vi "camera shutter.vi"() -> ()   [LabVIEW 2015]
doc: "Manually blink and LED attached to a digital output channel of a LINX device by clicking and LED control in LabVIEW."
uses:
  <vilib>/MakerHub/LINX/Public/Peripherals/Analog/Analog Read 1 Chan.vi
  <vilib>/MakerHub/LINX/Public/Peripherals/Digital/Digital Write N Chans.vi
  <vilib>/MakerHub/LINX/LMH-LINX.lvlib
panel:
  in  "Analog Channel":u8
  in  "OK Button":bool
  out "Loop Rate (Hz)":u32
  in  "Serial Port":refnum<visa-resource-name>
  in  "Stop Button":bool
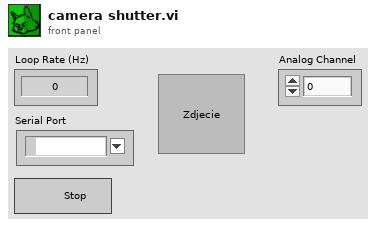
[diagram p1: front panel]
types:
  T1 = typedef "LMH-LINX.lvlib/LINX Ref.ctl" = cluster{"Platform":T2, "Interface":T3, "LINX Device Config":T4}
  T2 = typedef "LMH-LINX.lvlib/Platform.ctl" = enum16{"LINX", "myRIO"}
  T3 = typedef "LMH-LINX.lvlib/Interface.ctl" = enum16{"Serial", "TCP"}
  T4 = typedef "LMH-LINX.lvlib/Device.lvlib/LINX Device Config.ctl" = cluster{"Interface":T3, "COM Port":refnum<visa-resource-name>, "TCP Configuration":T5, "Device Family":u8, "Device ID":u8, "Device Name":string, "TCP Ref":refnum<k5>, "Channels":T6}
  T5 = typedef "LMH-LINX.lvlib/Device.lvlib/TCP Config.ctl" = cluster{"IP Address":string, "Port":u16}
  T6 = typedef "LMH-LINX.lvlib/Channels.ctl" = cluster{"DI":u8[], "DO":u8[], "AI":u8[], "AO":u8[], "PWM":u8[], "QE":u8[], "UART":u8[], "I2C 2":u8[], "SPI":u8[], "CAN":u8[], "Servo":u8[], "AI Ref (V)":dbl, "AO Ref (V)":dbl, "AO Resolution (Bits)":u8}
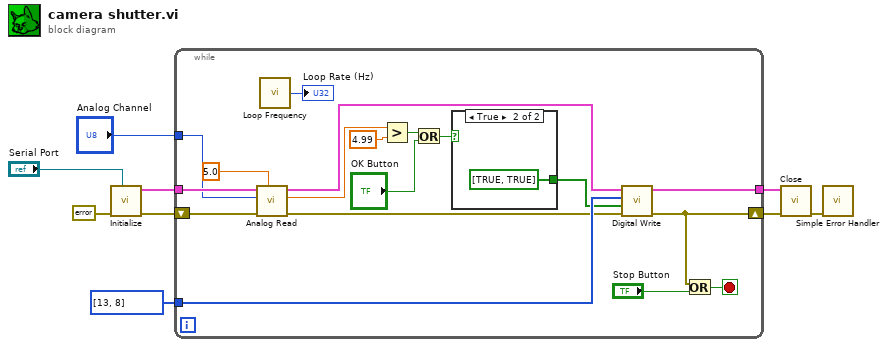
[diagram p0: block diagram]
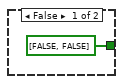
[diagram p2: hidden frame]
diagram:
  n1 = call <vilib>:"Initialize.vi"("Serial Port"="Serial Port", "Error In"=errorcluster {"status"=FALSE, "code"=0, "source"=""}) -> ("Error Out"=w8:errorcluster, "LINX Ref"=w9:T1)  [unwired: 7 in, 1 out]
  n2 = while {
    tunnel: w9 -> [w20]
    tunnel: [w25] -> w7
    shift-right: [w24] -> w6
    shift-left: w8 -> [w19]
    tunnel: u8[] [13, 8] ("DO Channels") -> [w22]
    tunnel: "Analog Channel" -> [w16]
    stop <- w27 stop-if-true
    n3 = call-poly <vilib>:"Analog Read.vi"("AI Range (V)"=5.0, "Error In"=w19, "Analog Channel"=w16, "LINX Resource"=w20) -> ("Error Out"=w17:errorcluster, "AI Value"=w10:dbl, "LINX Resource"=w18:T1)  [unwired: 4 in, 1 out]
    n4 = call <vilib>:"Loop Frequency.vi"() -> ("Loop Rate (Hz)"=→"Loop Rate (Hz)":u32)
    n5 = Greater?(x=w10, y=4.99) -> (0:w11:bool)
    n6 = Or(x=w11, y="OK Button") -> (x .or. y?=w12:bool)
    n7 = case shown="True" w12 {
      tunnel: [bool[] [FALSE, FALSE] ("Values") bool[] [TRUE, TRUE] ("Values")] -> w21
      frame False {
      }
      frame True {
      }
    }
    n8 = call-poly <vilib>:"Digital Write.vi"("Error In"=w17, "Values"=w21, "DO Channels"=w22, "LINX Resource"=w18) -> ("Error Out"=w24:errorcluster, "LINX Resource"=w25:T1)  [unwired: 6 in]
    n9 = Or(x=w24, y="Stop Button") -> (x .or. y?=w27:bool)
  }
  n10 = call <vilib>:"Close.vi"("Error In"=w6, "LINX Resource"=w7) -> ("Error Out"=w4:errorcluster)  [unwired: 8 in, 1 out]
  n11 = call <vilib>:"Simple Error Handler.vi"("error in (no error)"=w4) -> ()  [unwired: 4 in, 5 out]
